vi "Delete Standard Header.vi"(8 "error in (no error)":errorcluster, 11 "Save Image in":refnum<class "Save Image.lvclass">) -> (0 "error out":errorcluster, 3 "Save Image out":refnum<class "Save Image.lvclass">)   [LabVIEW 2018, in "Save Image.lvclass"]
uses:
  Save Image.lvclass
  Save Image.lvclass/Save Image.ctl
  Header/Header.lvclass
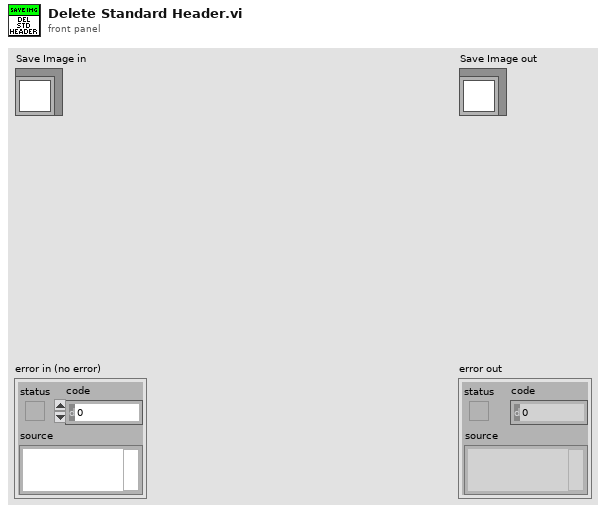
[diagram p1: front panel]
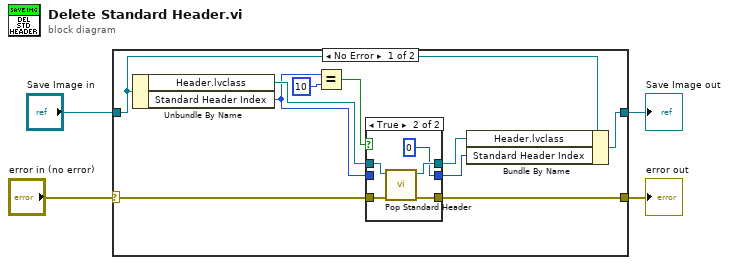
[diagram p0: block diagram]
diagram:
  n1 = case shown="No Error" "error in (no error)" {
    selector: "error in (no error)" -> [w7 w24]
    tunnel: [w8 w24] -> w3
    tunnel: [w10 w23] -> w1
    tunnel: "Save Image in" -> [w11 w23]
    frame No Error {
      n2 = Unbundle By Name(w11) -> ("Header.lvclass"=w12:refnum<class "Header.lvclass">, "Standard Header Index"=w5:u8)
      n3 = Equal?(x=w5, y=10) -> (x = y?=w13:bool)
      n4 = case shown="True" w13 {
        tunnel: w12 -> [w17 w22]
        tunnel: [w17 w21] -> w9
        tunnel: [w16 w20] -> w8
        tunnel: w7 -> [w16 w19]
        tunnel: [w15 u8 0] -> w6
        tunnel: w5 -> [w15 _]
        frame False {
        }
        frame True {
          n5 = call "Pop Standard Header.vi"("error in (no error)"=w19, "Header in"=w22) -> ("error out"=w20:errorcluster, "Header out"=w21:refnum<class "Header.lvclass">)  [unwired: 7 in, 1 out]
        }
      }
      n6 = Bundle By Name(cluster=w11, "Header.lvclass"=w9, "Standard Header Index"=w6) -> (w10:refnum<class "Save Image.lvclass">)
    }
    frame Error {
    }
  }
  "error out" <- w3
  "Save Image out" <- w1
